vi "Example Callback - PositionReached Callback.vi"(4 "PositionReached":refnum<user-event>, 5 "Event Data":cluster{"sender":refnum<k24>, "position":i32}, 6 "Control Ref":refnum<k24>, 7 "Event Common Data":T1) -> ()   [LabVIEW 2013]
uses:
  C:/tf/play/labview/Tinkerforge.dll
  Tinkerforge.dll
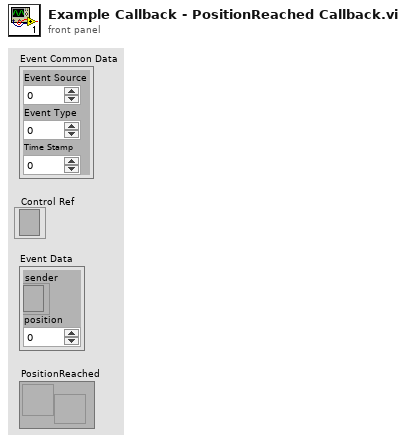
[diagram p1: front panel]
types:
  T1 = cluster{"Event Source":i32, "Event Type":u32, "Time Stamp":u32}
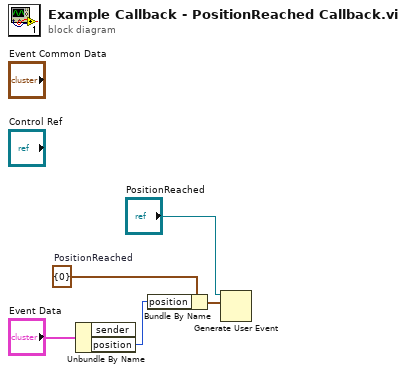
[diagram p0: block diagram]
diagram:
  w4 = cluster{"position":i32} {"position"=0}  # PositionReached
  n1 = Unbundle By Name("Event Data") -> ("position"=w3:i32)  [unwired: 1 out]
  n2 = Bundle By Name(cluster=w4, "position"=w3) -> (w2:cluster{"position":i32})
  n3 = Generate User Event(user event="PositionReached", event data cluster=w2) -> ()  [unwired: 2 in, 2 out]
